vi "Periodic Tasks.vi"(8 "error in":errorcluster) -> ()   [LabVIEW 2015]
doc: "This VI runs in parallel to other tasks. It can contain as many user-defined periodic loops as you need. These can carry out PID or other sorts of timed response."
uses:
  Type Defs/Shooter State.ctl
  Type Defs/Intake State.ctl
  Type Defs/Porticullis State.ctl
  <vilib>/Rock Robotics/WPI/Solenoid/WPI_SolenoidValue.ctl
  <vilib>/Rock Robotics/WPI/DriverStation/WPI_DriverStationRobotMode2.ctl
  <vilib>/Rock Robotics/WPI/Relay/WPI_RelayValue.ctl
  Robot Global Data.vi
  <vilib>/Rock Robotics/WPI/Utilities/WPI_GetSetVariantRefNum.vi
  <vilib>/Rock Robotics/WPI/Solenoid/WPI_SolenoidSetEnum.vi
  <vilib>/addons/control/pid/pid.llb/PID (DBL).vi
  <vilib>/addons/control/pid/NI_PID_pid.lvlib
panel:
  in  "Numeric 2":dbl=1.0 format="%#_13g"
  in  "Numeric":dbl=1.0 format="%#_13g"
  out "Arm Deegres":dbl
  out "Gauge":dbl(knob) scale=0.0..10.0
  in  "Stall Speed":dbl=-0.3
  in  "Setpoint Intake 1":dbl=81.0 format="%#_13g"
  in  "Setpoint intake":dbl=81.0 format="%#_13g"
  in  "X*50 = s":dbl=30.0 format="%#_13g"
  # "78 - intake ball"
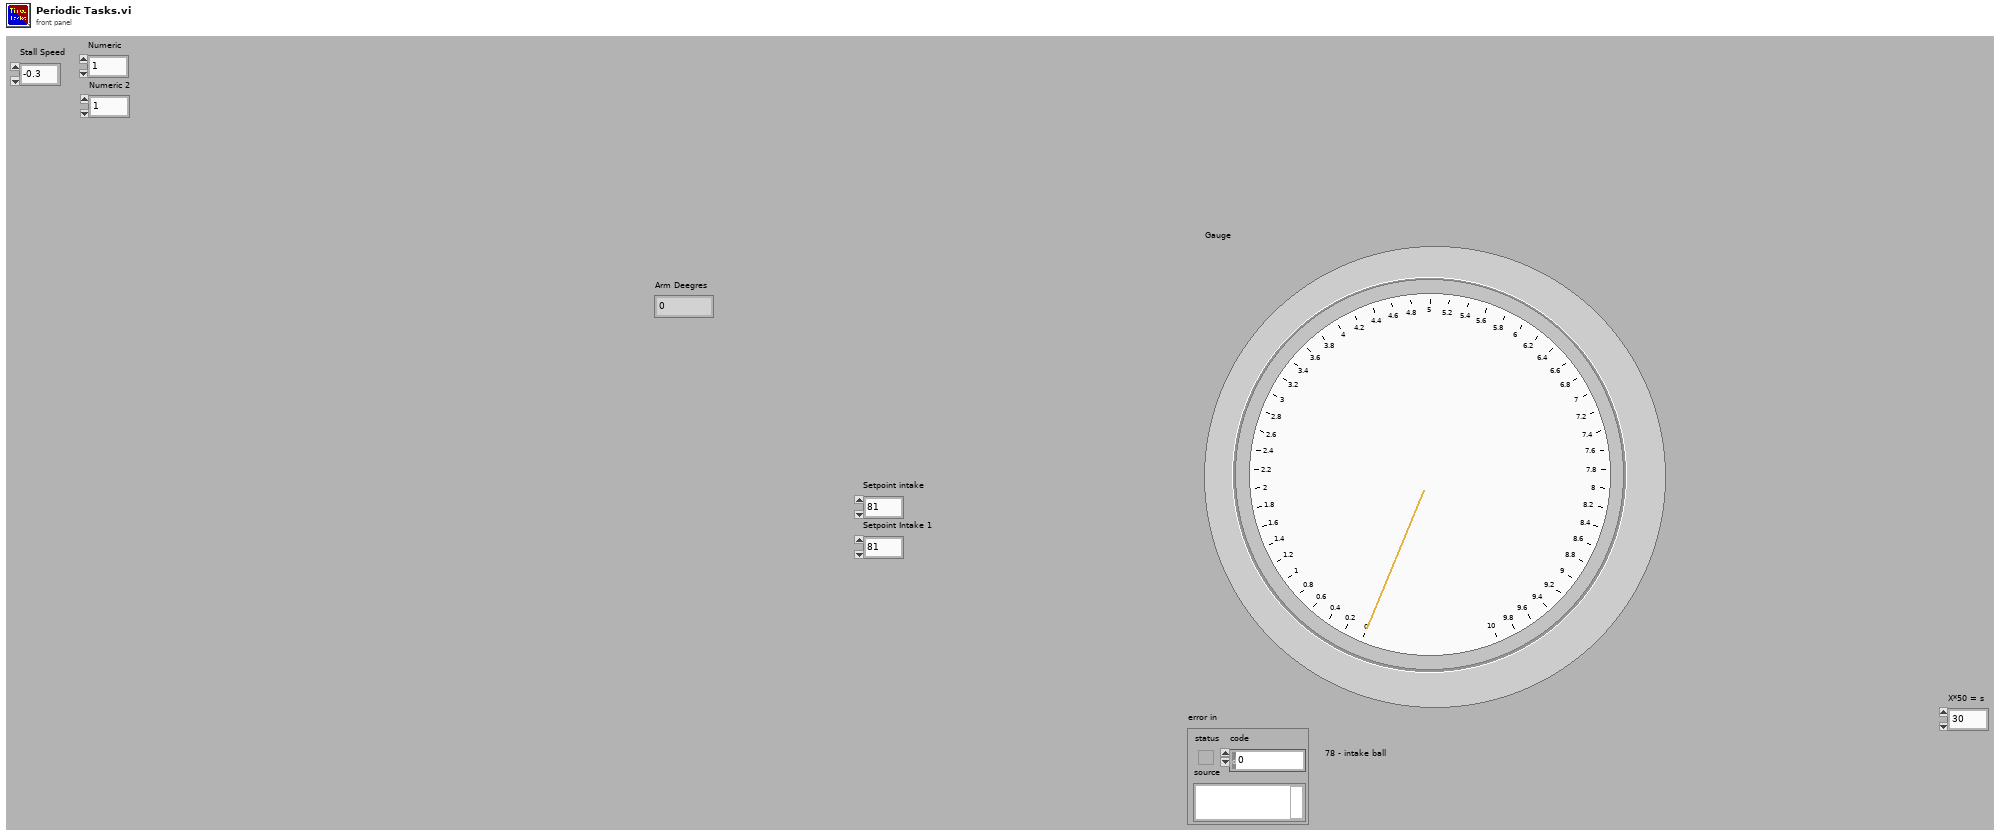
[diagram p1: front panel]
types:
  T1 = typedef "Porticullis State.ctl" = enum16{"Wait position", "Back up", "Reset Encoder", "Go Forward", "Finished"}
  T2 = typedef "Intake State.ctl" = enum16{"Resting", "Intake position", "Track Forward", "Raise Arm", "Track Reverse", "Defense position", "Armless Intake", "Cross Porticullis"}
  T3 = typedef "Shooter State.ctl" = enum16{"Resting", "Start Shooter", "Shooooot!"}
  T4 = typedef "WPI_RobotDriveDevRef.ctl" = cluster{"DevStatus":errorcluster, "Motors[]":T5[], "Square Inputs":bool, "Max Output":dbl}
  T5 = typedef "WPI_MotorControlDeviceRef.ctl" = cluster{"DeviceStatus":errorcluster, "Type":T6, "PWM":cluster{"PWM Channel":T7, "DeadBand":T8}, "CAN":cluster{"Device Number":u8, "Control Mode":T9, "Semaphore":T10, "Max Vout":dbl, "TalonSRX Control Mode":T11}, "Invert":bool}
  T6 = typedef "WPI_MotorControlType.ctl" = enum16{"PWM", "CAN", "CANTalonSRX"}
  T7 = typedef "FPGA_DIOPWMChannel.ctl" = enum8{"PWM 0", "PWM 1", "PWM 2", "PWM 3", "PWM 4", "PWM 5", "PWM 6", "PWM 7", "PWM 8", "PWM 9", "PWM MXP 0", "PWM MXP 1", "PWM MXP 2", "PWM MXP 3", "PWM MXP 4", "PWM MXP 5", "PWM MXP 6", "PWM MXP 7", "PWM MXP 8", "PWM MXP 9", "Invalid"}
  T8 = typedef "WPI_PWMDeadband.ctl" = cluster{"Name":string, "maxPositivePwm":i32, "minPositivePwm":i32, "centerPwm":i32, "maxNegativePwm":i32, "minNegativePwm":i32, "angularRange":u16}
  T9 = typedef "WPI_CANJaguar_ControlMode.ctl" = enum8{"Percent VBus", "Current", "Speed", "Position", "Voltage"}
  T10 = typedef "Semaphore RefNum" = refnum<k1>
  T11 = typedef "WPI_CANTalonSRX_APIControlMode.ctl" = enum8{"Percent VBus", "Speed", "Position", "Slave", "Unchanged / Invalid", "Voltage Compensation", "Current", "Motion Profile"}
  T12 = typedef "WPI_EncoderDevRef.ctl" = cluster{"DevStatus":errorcluster, "EncoderIndex":T13, "CounterIndex":T14, "DistancePerCount":dbl, "Decoding Type":T15}
  T13 = typedef "FPGA_EncoderIdx.ctl" = enum8{"Enc 0", "Enc 1", "Enc 2", "Enc 3", "Enc 4", "Enc 5", "Enc 6", "Enc 7", "Invalid"}
  T14 = typedef "FPGA_CounterCtrSystemIndex.ctl" = enum8{"Ctr 0", "Ctr 1", "Ctr 2", "Ctr 3", "Ctr 4", "Ctr 5", "Ctr 6", "Ctr 7", "Invalid"}
  T15 = typedef "WPI_EncoderType.ctl" = enum16{"1x", "2x", "4x"}
  T16 = typedef "WPI_SolenoidDevRef.ctl" = cluster{"DevStatus":errorcluster, "Pneumatics Control Module":u8, "Forward Solenoid Channel":T17, "Reverse Solenoid Channel":T17}
  T17 = typedef "WPI_SolenoidChannel.ctl" = enum8{"Solenoid 0", "Solenoid 1", "Solenoid 2", "Solenoid 3", "Solenoid 4", "Solenoid 5", "Solenoid 6", "Solenoid 7", "Invalid"}
  T18 = typedef "WPI_RelayValue.ctl" = enum16{"Off", "On", "Forward", "Reverse"}
  T19 = typedef "WPI_DriverStationRobotMode2.ctl" = enum16{"Autonomous Disabled", "Autonomous Enabled", "Teleop Disabled", "Teleop Enabled", "Disconnected", "Finish", "Test Disabled", "Test Enabled", "Emergency Stopped"}
  T20 = typedef "WPI_SolenoidValue.ctl" = enum16{"Off", "On", "Forward", "Reverse"}
  T21 = typedef "WPI_RelayDevRef.ctl" = cluster{"DevStatus":errorcluster, "Relay Channel":T22, "Relay Direction":T23}
  T22 = typedef "FPGA_DIORelayChannel.ctl" = enum8{"Relay 0", "Relay 1", "Relay 2", "Relay 3", "Invalid"}
  T23 = typedef "WPI_RelayDirection.ctl" = enum16{"Both directions", "Forward only", "Reverse only"}
  T24 = typedef "WPI_DigitalInputDevRef.ctl" = cluster{"DevStatus":errorcluster, "DIO Channel":T25}
  T25 = typedef "FPGA_DIOChannel.ctl" = enum8{"DIO 0", "DIO 1", "DIO 2", "DIO 3", "DIO 4", "DIO 5", "DIO 6", "DIO 7", "DIO 8", "DIO 9", "DIO MXP 0", "DIO MXP 1", "DIO MXP 2", "DIO MXP 3", "DIO MXP 4", "DIO MXP 5", "DIO MXP 6", "DIO MXP 7", "DIO MXP 8", "DIO MXP 9", "DIO MXP 10", "DIO MXP 11", "DIO MXP 12", "DIO MXP 13", "DIO MXP 14", "DIO MXP 15", "Invalid"}
  T26 = typedef "WPI_SwitchDevRef.ctl" = cluster{"DevStatus":errorcluster, "DIO Channel":T25, "CntIndex":T14, "Normally Closed":bool}
  T27 = cluster{"proportional gain (Kc)":dbl, "integral time (Ti, min)":dbl, "derivative time (Td, min)":dbl}
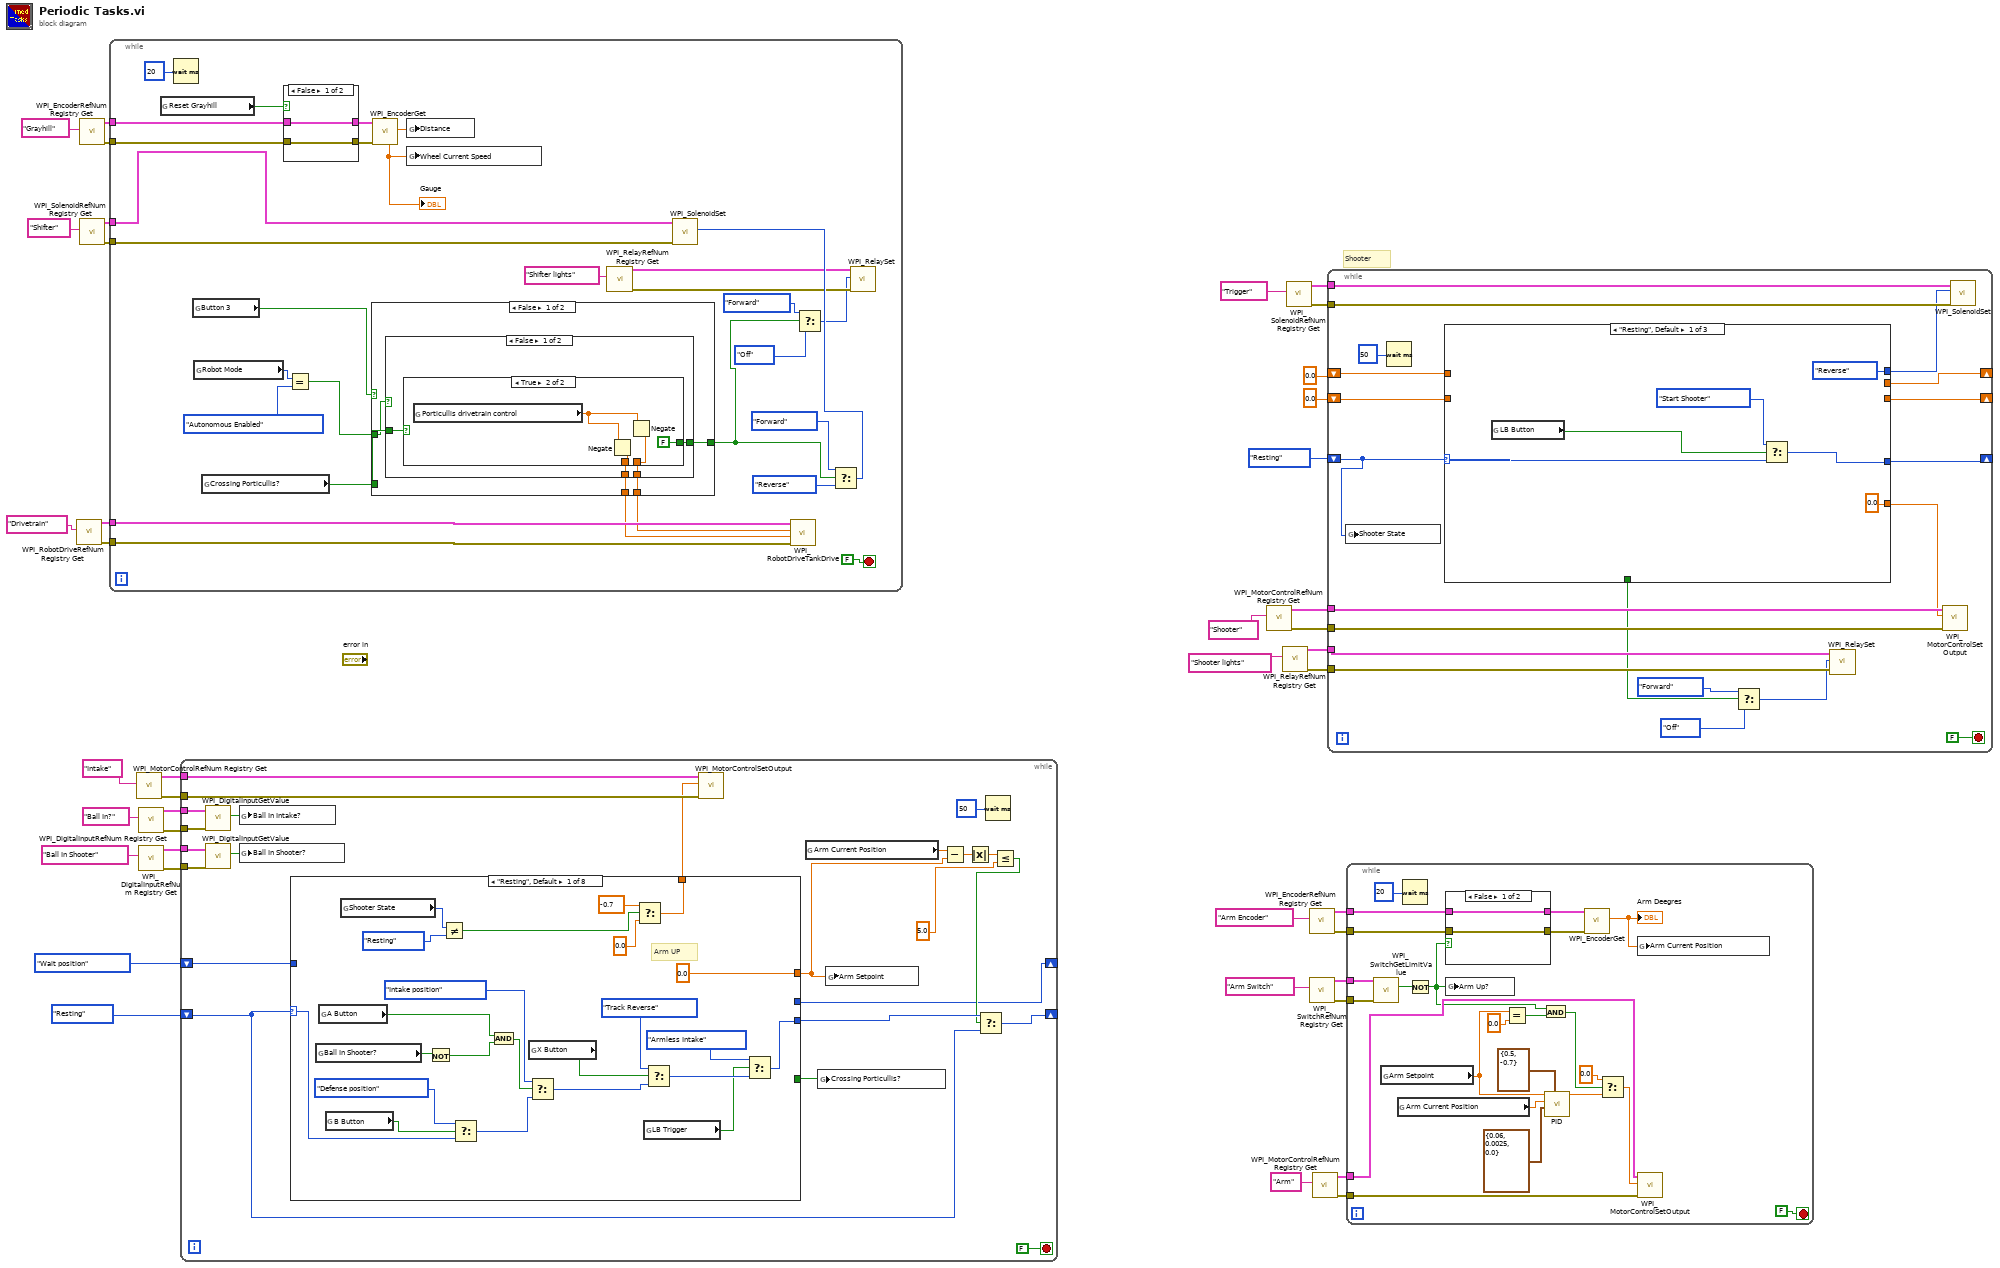
[diagram p0: block diagram]
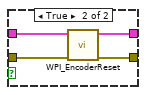
[diagram p2: hidden frame]
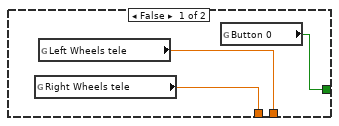
[diagram p3: hidden frame]
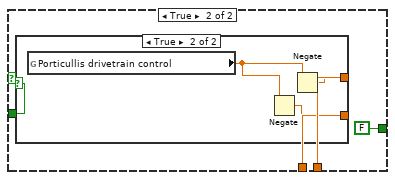
[diagram p4: hidden frame]
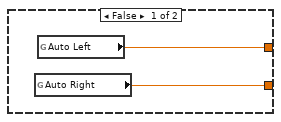
[diagram p5: hidden frame]
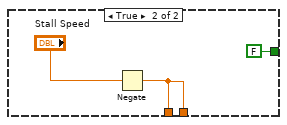
[diagram p6: hidden frame]
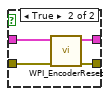
[diagram p7: hidden frame]
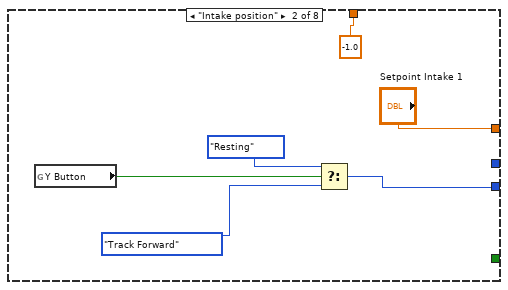
[diagram p8: hidden frame]
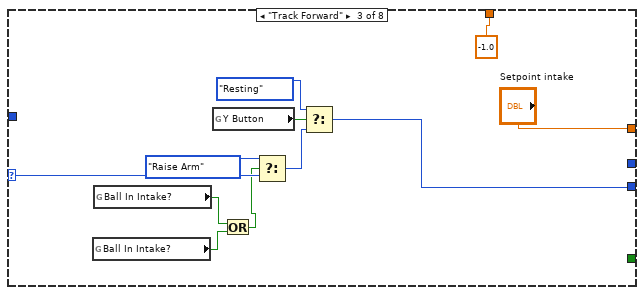
[diagram p9: hidden frame]
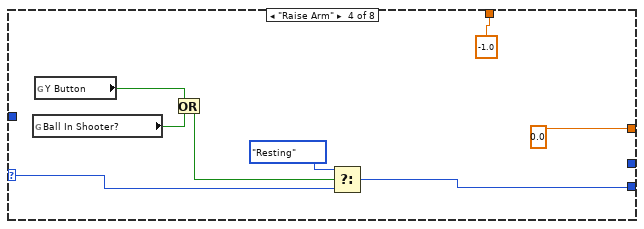
[diagram p10: hidden frame]
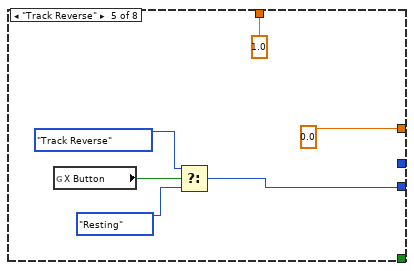
[diagram p11: hidden frame]
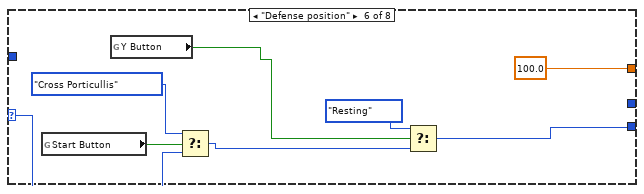
[diagram p12: hidden frame]
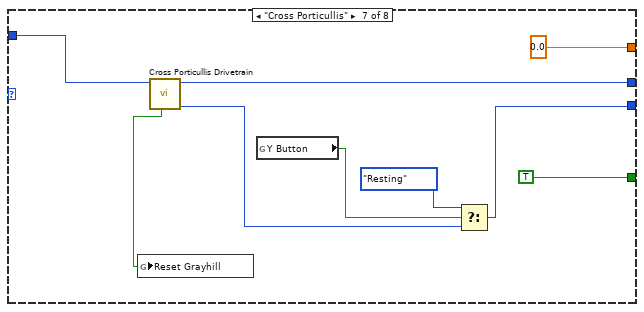
[diagram p13: hidden frame]
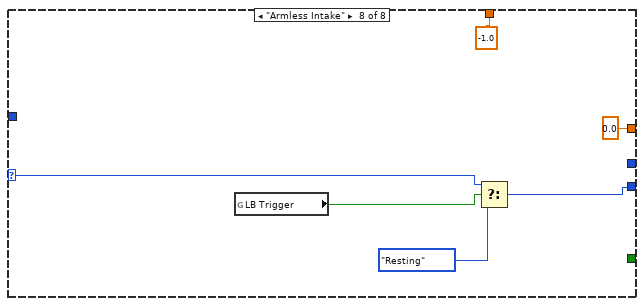
[diagram p14: hidden frame]
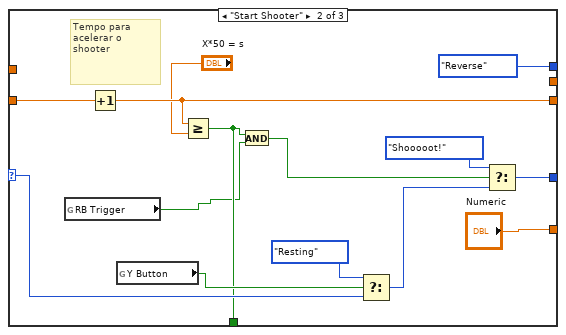
[diagram p15: hidden frame]
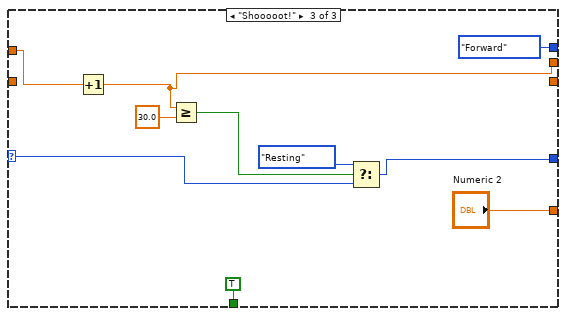
[diagram p16: hidden frame]
diagram:
  # "Shooter"
  n1 = call <vilib>:"WPI_RobotDriveRefNum Registry Get.vi"("refnum name"="Drivetrain") -> ("error out"=w13:errorcluster, "RobotDriveDevRef"=w14:T4)  [unwired: 9 in]
  n2 = call <vilib>:"WPI_EncoderRefNum Registry Get.vi"("refnum name"="Grayhill") -> ("error out"=w16:errorcluster, "EncoderDevRef"=w17:T12)  [unwired: 9 in]
  n3 = call <vilib>:"WPI_SolenoidRefNum Registry Get.vi"("refnum name"="Shifter") -> ("error out"=w21:errorcluster, "SolenoidDevRef"=w20:T16)  [unwired: 9 in]
  n4 = while {
    tunnel: w20 -> [w69]
    tunnel: w21 -> [w68]
    tunnel: w17 -> [w65]
    tunnel: w16 -> [w64]
    tunnel: w14 -> [w59]
    tunnel: w13 -> [w58]
    stop <- FALSE stop-if-true
    n5 = global read "Robot Global Data.vi" "Reset Grayhill"() -> (w53:bool)
    n6 = Wait (ms)(milliseconds to wait=u32 20) -> ()  [unwired: 1 out]
    n7 = global read "Robot Global Data.vi" "Button 3"() -> (w49:bool)
    n8 = global read "Robot Global Data.vi" "Robot Mode"() -> (w52:T19)
    n9 = global read "Robot Global Data.vi" "Crossing Porticullis?"() -> (w57:bool)
    n10 = case shown="False" w53 {
      tunnel: [w100 w105] -> w66
      tunnel: [w101 w104] -> w67
      tunnel: w65 -> [w100 w103]
      tunnel: w64 -> [w101 w102]
      frame False {
      }
      frame True {
        n11 = call <vilib>:"WPI_EncoderReset.vi"("error in (no error)"=w102, "EncoderDevRef"=w103) -> ("error out"=w104:errorcluster, "EncoderDevRef"=w105:T12)  [unwired: 8 in]
      }
    }
    n12 = Equal?(x=w52, y=WPI_DriverStationRobotMode2."Autonomous Enabled") -> (x = y?=w50:bool)
    n13 = case shown="False" w49 {
      tunnel: w57 -> [w76 _]
      tunnel: [w75 w97] -> w56
      tunnel: [w74 w97] -> w55
      tunnel: [w73 FALSE ("Button 0")] -> w43
      tunnel: w50 -> [w72 _]
      frame False {
        n14 = case shown="False" w72 {
          tunnel: w76 -> [w80 w88]
          tunnel: [w79 w90] -> w75
          tunnel: [w78 w91] -> w74
          tunnel: [w77 FALSE ("Button 0")] -> w73
          frame False {
            n15 = case shown="True" w80 {
              tunnel: [w83 w85] -> w79
              tunnel: [w82 w86] -> w78
              tunnel: [w81 FALSE ("Button 0")] -> w77
              frame False {
                n16 = global read "Robot Global Data.vi" "Right Wheels tele"() -> (w83:dbl)
                n17 = global read "Robot Global Data.vi" "Left Wheels tele"() -> (w82:dbl)
                n18 = global read "Robot Global Data.vi" "Button 0"() -> (w81:bool)
              }
              frame True {
                n19 = global read "Robot Global Data.vi" "Porticullis drivetrain control"() -> (w87:dbl)
                n20 = Negate(x=w87) -> (-x=w85:dbl)
                n21 = Negate(x=w87) -> (-x=w86:dbl)
              }
            }
          }
          frame True {
            n22 = case shown="True" w88 {
              tunnel: [w93 w94] -> w91
              tunnel: [w92 w95] -> w90
              frame False {
                n23 = global read "Robot Global Data.vi" "Auto Right"() -> (w92:dbl)
                n24 = global read "Robot Global Data.vi" "Auto Left"() -> (w93:dbl)
              }
              frame True {
                n25 = global read "Robot Global Data.vi" "Porticullis drivetrain control"() -> (w96:dbl)
                n26 = Negate(x=w96) -> (-x=w95:dbl)
                n27 = Negate(x=w96) -> (-x=w94:dbl)
              }
            }
          }
        }
      }
      frame True {
        n28 = Negate(x="Stall Speed") -> (-x=w97:dbl)
      }
    }
    n29 = call <vilib>:"WPI_EncoderGet.vi"("error in (no error)"=w67, "EncoderDevRef"=w66) -> ("Distance"=w63:dbl, "Rate"=w60:dbl)  [unwired: 4 in, 4 out]
    "Gauge" <- w60
    n30 = global write "Robot Global Data.vi" "Distance"(w63) -> ()
    n31 = global write "Robot Global Data.vi" "Wheel Current Speed"(w60) -> ()
    n32 = call <vilib>:"WPI_RelayRefNum Registry Get.vi"("refnum name"="Shifter lights") -> ("error out"=w47:errorcluster, "RelayDevRef"=w48:T21)  [unwired: 9 in]
    n33 = call <vilib>:"WPI_RobotDriveTankDrive.vi"("error in (no error)"=w58, "Right axis value"=w56, "Left axis value"=w55, "RobotDriveDevRef"=w59) -> ()  [unwired: 5 in, 3 out]
    n34 = Select(t=WPI_RelayValue."Forward" ("RelayValue"), s=w43, f=WPI_RelayValue."Off" ("RelayValue")) -> (s? t:f=w45:T18)
    n35 = Select(t=WPI_SolenoidValue."Forward" ("Value"), s=w43, f=WPI_SolenoidValue."Reverse" ("Value")) -> (s? t:f=w54:T20)
    n36 = call-poly <vilib>:"WPI_SolenoidSet.vi"("error in (no error)"=w68, "Value"=w54, "SolenoidDevRef"=w69) -> ()  [unwired: 7 in, 2 out]
    n37 = call <vilib>:"WPI_RelaySet.vi"("error in (no error)"=w47, "RelayValue"=w45, "RelayDevRef"=w48) -> ()  [unwired: 7 in, 2 out]
  }
  n38 = call <vilib>:"WPI_MotorControlRefNum Registry Get.vi"("refnum name"="Intake") -> ("error out"=w29:errorcluster, "MotorControlDevRef"=w30:T5)  [unwired: 9 in]
  n39 = call <vilib>:"WPI_DigitalInputRefNum Registry Get.vi"("refnum name"="Ball In?") -> ("error out"=w27:errorcluster, "DigitalInputDevRef"=w28:T24)  [unwired: 9 in]
  n40 = call <vilib>:"WPI_DigitalInputRefNum Registry Get.vi"("refnum name"="Ball In Shooter") -> ("error out"=w25:errorcluster, "DigitalInputDevRef"=w26:T24)  [unwired: 9 in]
  n41 = while {
    shift-right: [w124] -> _
    shift-left: Intake_State."Resting" -> [w109]
    tunnel: w30 -> [w127]
    tunnel: w29 -> [w126]
    tunnel: w28 -> [w119]
    tunnel: w27 -> [w118]
    tunnel: w26 -> [w117]
    tunnel: w25 -> [w116]
    shift-right: [w106] -> _
    shift-left: Porticullis_State."Wait position" -> [w108]
    stop <- FALSE stop-if-true
    n42 = call <vilib>:"WPI_DigitalInputGetValue.vi"("error in (no error)"=w118, "DigitalInputDevRef"=w119) -> ("Value"=w121:bool)  [unwired: 7 in, 2 out]
    n43 = call <vilib>:"WPI_DigitalInputGetValue.vi"("error in (no error)"=w116, "DigitalInputDevRef"=w117) -> ("Value"=w120:bool)  [unwired: 7 in, 2 out]
    n44 = global write "Robot Global Data.vi" "Ball In Intake?"(w121) -> ()
    n45 = global write "Robot Global Data.vi" "Ball In Shooter?"(w120) -> ()
    n46 = case shown="\"Resting\", Default" w109 {
      selector: w109 -> [w134 _ w167 w175 _ w185 _ w202]
      tunnel: [w145 -1.0 ("f") -1.0 -1.0 1.0 ("f") _ _ -1.0 ("f")] -> w125
      tunnel: [0.0 "Setpoint Intake 1" "Setpoint intake" 0.0 0.0 100.0 0.0 0.0 ("Setpoint intake")] -> w107
      tunnel: [w131 w154 w163 w174 w180 w187 w195 w204] -> w123
      tunnel: [_ _ _ _ _ _ TRUE ("Crossing Porticullis?") _] -> w110
      tunnel: w108 -> [_ _ _ _ _ _ w197 _]
      tunnel: [_ _ _ _ _ _ w196 _] -> w106
      frame "Resting", Default {
        # "Arm UP"
        n47 = global read "Robot Global Data.vi" "Ball In Shooter?"() -> (w149:bool)
        n48 = global read "Robot Global Data.vi" "A Button"() -> (w147:bool)
        n49 = global read "Robot Global Data.vi" "B Button"() -> (w133:bool)
        n50 = global read "Robot Global Data.vi" "Shooter State"() -> (w143:T3)
        n51 = Not(x=w149) -> (.not. x?=w148:bool)
        n52 = Not Equal?(x=w143, y=Shooter_State."Resting" ("t")) -> (x != y?=w142:bool)
        n53 = Select(t=Intake_State."Defense position", s=w133, f=w134) -> (s? t:f=w136:T2)
        n54 = And(x=w147, y=w148) -> (x .and. y?=w146:bool)
        n55 = global read "Robot Global Data.vi" "X Button"() -> (w137:bool)
        n56 = Select(t=Intake_State."Intake position", s=w146, f=w136) -> (s? t:f=w139:T2)
        n57 = Select(t=-0.7, s=w142, f=0.0) -> (s? t:f=w145:dbl)
        n58 = global read "Robot Global Data.vi" "LB Trigger"() -> (w129:bool)
        n59 = Select(t=Intake_State."Track Reverse", s=w137, f=w139) -> (s? t:f=w132:T2)
        n60 = Select(t=Intake_State."Armless Intake", s=w129, f=w132) -> (s? t:f=w131:T2)
      }
      frame "Intake position" {
        n61 = global read "Robot Global Data.vi" "Y Button"() -> (w152:bool)
        n62 = Select(t=Intake_State."Resting", s=w152, f=Intake_State."Track Forward") -> (s? t:f=w154:T2)
      }
      frame "Track Forward" {
        n63 = global read "Robot Global Data.vi" "Ball In Intake?"() -> (w160:bool)
        n64 = global read "Robot Global Data.vi" "Ball In Intake?"() -> (w159:bool)
        n65 = global read "Robot Global Data.vi" "Y Button"() -> (w161:bool)
        n66 = Or(x=w159, y=w160) -> (x .or. y?=w158:bool)
        n67 = Select(t=Intake_State."Raise Arm", s=w158, f=w167) -> (s? t:f=w164:T2)
        n68 = Select(t=Intake_State."Resting", s=w161, f=w164) -> (s? t:f=w163:T2)
      }
      frame "Raise Arm" {
        n69 = global read "Robot Global Data.vi" "Ball In Shooter?"() -> (w171:bool)
        n70 = global read "Robot Global Data.vi" "Y Button"() -> (w170:bool)
        n71 = Or(x=w170, y=w171) -> (x .or. y?=w169:bool)
        n72 = Select(t=Intake_State."Resting", s=w169, f=w175) -> (s? t:f=w174:T2)
      }
      frame "Track Reverse" {
        n73 = global read "Robot Global Data.vi" "X Button"() -> (w179:bool)
        n74 = Select(t=Intake_State."Track Reverse", s=w179, f=Intake_State."Resting" ("t")) -> (s? t:f=w180:T2)
      }
      frame "Defense position" {
        n75 = global read "Robot Global Data.vi" "Start Button"() -> (w183:bool)
        n76 = global read "Robot Global Data.vi" "Y Button"() -> (w188:bool)
        n77 = Select(t=Intake_State."Cross Porticullis", s=w183, f=w185) -> (s? t:f=w186:T2)
        n78 = Select(t=Intake_State."Resting", s=w188, f=w186) -> (s? t:f=w187:T2)
      }
      frame "Cross Porticullis" {
        n79 = call "Cross Porticullis Drivetrain.vi"("Local in"=w197) -> ("Global Machine"=w194:T2, "Local Machine"=w196:T1, "Reset Enconder"=w191:bool)  [unwired: 8 in]
        n80 = global write "Robot Global Data.vi" "Reset Grayhill"(w191) -> ()
        n81 = global read "Robot Global Data.vi" "Y Button"() -> (w192:bool)
        n82 = Select(t=Intake_State."Resting", s=w192, f=w194) -> (s? t:f=w195:T2)
      }
      frame "Armless Intake" {
        n83 = global read "Robot Global Data.vi" "LB Trigger"() -> (w205:bool)
        n84 = Select(t=w202, s=w205, f=Intake_State."Resting" ("t")) -> (s? t:f=w204:T2)
      }
    }
    n85 = call <vilib>:"WPI_MotorControlSetOutput.vi"("error in (no error)"=w126, "Output"=w125, "MotorControlDevRef"=w127) -> ()  [unwired: 6 in, 3 out]
    n86 = global read "Robot Global Data.vi" "Arm Current Position"() -> (w115:dbl)
    n87 = global write "Robot Global Data.vi" "Crossing Porticullis?"(w110) -> ()
    n88 = global write "Robot Global Data.vi" "Arm Setpoint"(w107) -> ()
    n89 = Subtract(x=w115, y=w107) -> (x-y=w114:dbl)
    n90 = Absolute Value(x=w114) -> (abs(x)=w113:dbl)
    n91 = Wait (ms)(milliseconds to wait=u32 50) -> ()  [unwired: 1 out]
    n92 = Less Or Equal?(x=w113, y=5.0) -> (x <= y?=w111:bool)
    n93 = Select(t=w123, s=w111, f=w109) -> (s? t:f=w124:T2)
  }
  n94 = call <vilib>:"WPI_MotorControlRefNum Registry Get.vi"("refnum name"="Shooter") -> ("error out"=w36:errorcluster, "MotorControlDevRef"=w37:T5)  [unwired: 9 in]
  n95 = call <vilib>:"WPI_RelayRefNum Registry Get.vi"("refnum name"="Shooter lights") -> ("error out"=w1:errorcluster, "RelayDevRef"=w2:T21)  [unwired: 9 in]
  n96 = call <vilib>:"WPI_SolenoidRefNum Registry Get.vi"("refnum name"="Trigger") -> ("error out"=w33:errorcluster, "SolenoidDevRef"=w35:T16)  [unwired: 9 in]
  n97 = call <vilib>:"WPI_EncoderRefNum Registry Get.vi"("refnum name"="Arm Encoder") -> ("error out"=w4:errorcluster, "EncoderDevRef"=w5:T12)  [unwired: 9 in]
  n98 = call <vilib>:"WPI_SwitchRefNum Registry Get.vi"("refnum name"="Arm Switch") -> ("error out"=w6:errorcluster, "SwitchDevRef"=w7:T26)  [unwired: 9 in]
  n99 = call <vilib>:"WPI_MotorControlRefNum Registry Get.vi"("refnum name"="Arm") -> ("error out"=w11:errorcluster, "MotorControlDevRef"=w10:T5)  [unwired: 9 in]
  n100 = while {
    shift-right: [w220] -> _
    shift-left: Shooter_State."Resting" -> [w214]
    shift-right: [w218] -> _
    shift-left: 0.0 -> [w219]
    tunnel: w37 -> [w223]
    tunnel: w36 -> [w222]
    tunnel: w35 -> [w217]
    tunnel: w33 -> [w216]
    shift-right: [w212] -> _
    shift-left: 0.0 -> [w213]
    tunnel: w2 -> [w211]
    tunnel: w1 -> [w210]
    stop <- FALSE stop-if-true
    n101 = global write "Robot Global Data.vi" "Shooter State"(w214) -> ()
    n102 = Wait (ms)(milliseconds to wait=u32 50) -> ()  [unwired: 1 out]
    n103 = case shown="\"Resting\", Default" w214 {
      selector: w214 -> [w229 w237 w250]
      tunnel: [0.0 "Numeric" "Numeric 2"] -> w221
      tunnel: [w230 w241 w251] -> w220
      tunnel: w219 -> [_ w245 _]
      tunnel: [_ w244 _] -> w218
      tunnel: [WPI_SolenoidValue."Reverse" ("Value") WPI_SolenoidValue."Reverse" ("Value") WPI_SolenoidValue."Forward" ("Value")] -> w215
      tunnel: w213 -> [_ _ w247]
      tunnel: [_ _ w248] -> w212
      tunnel: [_ w233 TRUE] -> w209
      frame "Resting", Default {
        n104 = global read "Robot Global Data.vi" "LB Button"() -> (w226:bool)
        n105 = Select(t=Shooter_State."Start Shooter", s=w226, f=w229) -> (s? t:f=w230:T3)
      }
      frame "Start Shooter" {
        # "Tempo para acelerar o shooter"
        n106 = global read "Robot Global Data.vi" "RB Trigger"() -> (w232:bool)
        n107 = Increment(x=w245) -> (x+1=w244:dbl)
        n108 = global read "Robot Global Data.vi" "Y Button"() -> (w235:bool)
        n109 = Greater Or Equal?(x=w244, y="X*50 = s") -> (x >= y?=w233:bool)
        n110 = And(x=w233, y=w232) -> (x .and. y?=w240:bool)
        n111 = Select(t=Shooter_State."Resting", s=w235, f=w237) -> (s? t:f=w238:T3)
        n112 = Select(t=Shooter_State."Shooooot!", s=w240, f=w238) -> (s? t:f=w241:T3)
      }
      frame "Shooooot!" {
        n113 = Increment(x=w247) -> (x+1=w248:dbl)
        n114 = Greater Or Equal?(x=w248, y=30.0) -> (x >= y?=w252:bool)
        n115 = Select(t=Shooter_State."Resting", s=w252, f=w250) -> (s? t:f=w251:T3)
      }
    }
    n116 = Select(t=WPI_RelayValue."Forward" ("RelayValue"), s=w209, f=WPI_RelayValue."Off") -> (s? t:f=w206:T18)
    n117 = call <vilib>:"WPI_RelaySet.vi"("error in (no error)"=w210, "RelayValue"=w206, "RelayDevRef"=w211) -> ()  [unwired: 7 in, 2 out]
    n118 = call <vilib>:"WPI_MotorControlSetOutput.vi"("error in (no error)"=w222, "Output"=w221, "MotorControlDevRef"=w223) -> ()  [unwired: 6 in, 3 out]
    n119 = call-poly <vilib>:"WPI_SolenoidSet.vi"("error in (no error)"=w216, "Value"=w215, "SolenoidDevRef"=w217) -> ()  [unwired: 7 in, 2 out]
  }
  n120 = while {
    tunnel: w10 -> [w274]
    tunnel: w11 -> [w273]
    tunnel: w7 -> [w268]
    tunnel: w6 -> [w267]
    tunnel: w5 -> [w266]
    tunnel: w4 -> [w265]
    stop <- FALSE stop-if-true
    n121 = call <vilib>:"WPI_SwitchGetLimitValue.vi"("error in (no error)"=w267, "SwitchDevRef"=w268) -> ("Switch Pressed"=w264:bool)  [unwired: 7 in, 2 out]
    n122 = global read "Robot Global Data.vi" "Arm Setpoint"() -> (w263:dbl)
    n123 = global read "Robot Global Data.vi" "Arm Current Position"() -> (w272:dbl)
    n124 = Wait (ms)(milliseconds to wait=u32 20) -> ()  [unwired: 1 out]
    n125 = Not(x=w264) -> (.not. x?=w260:bool)
    n126 = case shown="False" w260 {
      tunnel: [w280 w284] -> w271
      tunnel: [w279 w283] -> w270
      tunnel: w266 -> [w280 w282]
      tunnel: w265 -> [w279 w281]
      frame False {
      }
      frame True {
        n127 = call <vilib>:"WPI_EncoderReset.vi"("error in (no error)"=w281, "EncoderDevRef"=w282) -> ("error out"=w283:errorcluster, "EncoderDevRef"=w284:T12)  [unwired: 8 in]
      }
    }
    n128 = global write "Robot Global Data.vi" "Arm Up?"(w260) -> ()
    n129 = Equal?(x=w263, y=0.0) -> (x = y?=w261:bool)
    n130 = And(x=w260, y=w261) -> (x .and. y?=w259:bool)
    n131 = call-poly <vilib>:"PID.vi"("output range"=cluster{"output high":dbl, "output low":dbl} {"output high"=0.5, "output low"=-0.7}, "PID gains"=T27 {"proportional gain (Kc)"=0.06, "integral time (Ti, min)"=0.0025, "derivative time (Td, min)"=0.0}, "process variable"=w272, "setpoint"=w263) -> ("output"=w257:dbl)  [unwired: 6 in, 1 out]
    n132 = call <vilib>:"WPI_EncoderGet.vi"("error in (no error)"=w270, "EncoderDevRef"=w271) -> ("Distance"=w269:dbl)  [unwired: 4 in, 5 out]
    "Arm Deegres" <- w269
    n133 = Select(t=0.0, s=w259, f=w257) -> (s? t:f=w256:dbl)
    n134 = global write "Robot Global Data.vi" "Arm Current Position"(w269) -> ()
    n135 = call <vilib>:"WPI_MotorControlSetOutput.vi"("error in (no error)"=w273, "Output"=w256, "MotorControlDevRef"=w274) -> ()  [unwired: 6 in, 3 out]
  }
